vi "ELVIS III v1.0 AO Enqueue Data.vi"(7 "AO Block Channels FPGA Reference":T1, 8 "error in (no error)":errorcluster, 11 "AO Block Write Configuration":T2={"AO FIFO Clock Divisor"=1000, "Wait Until Done?"=TRUE, "Write Mode"=0, "AO (N Samples) Configuration "=[]}) -> (0 "error out":errorcluster)   [LabVIEW 2021]
uses:
  <vilib>/myRIO/Common/Instrument Driver Framework/ELVIS III v1.0/AO Block/typedefs/ELVIS III AO Block Configuration.ctl
  <vilib>/myRIO/Common/Instrument Driver Framework/ELVIS III v1.0/AO Block/typedefs/ELVIS III AO Block Bank Data.ctl
  <vilib>/myRIO/Common/Instrument Driver Framework/ELVIS III v1.0/AO Block/typedefs/ELVIS III AO Block Channels FPGA Reference.ctl
  <vilib>/rvi/errors/niLvFpgaAdjustHostInterfaceError.vi
  <vilib>/rvi/interface/nirviReadWriteControl/nirviReadWriteControl.xnode
  NiFpgaLv.dll
  <vilib>/rvi/interface/Simulation/niFpgaSimulationCallBeginRW.vi
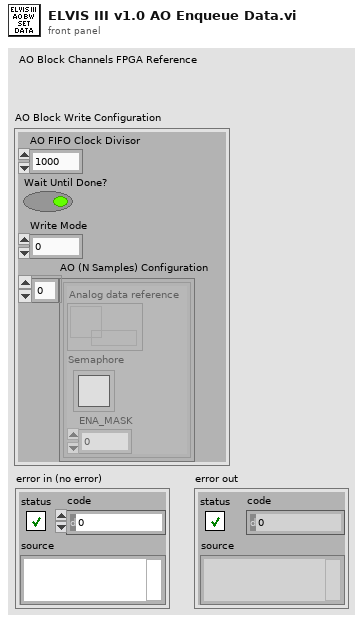
[diagram p1: front panel]
types:
  T1 = typedef "ELVIS III AO Block Channels FPGA Reference.ctl" = refnum<k20>
  T2 = typedef "ELVIS III AO Block Configuration.ctl" = cluster{"AO FIFO Clock Divisor":u32, "Wait Until Done?":bool, "Write Mode":u8, "AO (N Samples) Configuration ":T3[]}
  T3 = typedef "ELVIS III AO Block Bank Data.ctl" = cluster{"Analog data reference":refnum<data-value>, "Semaphore":T4, "ENA_MASK":u8}
  T4 = typedef "Semaphore RefNum" = refnum<k1>
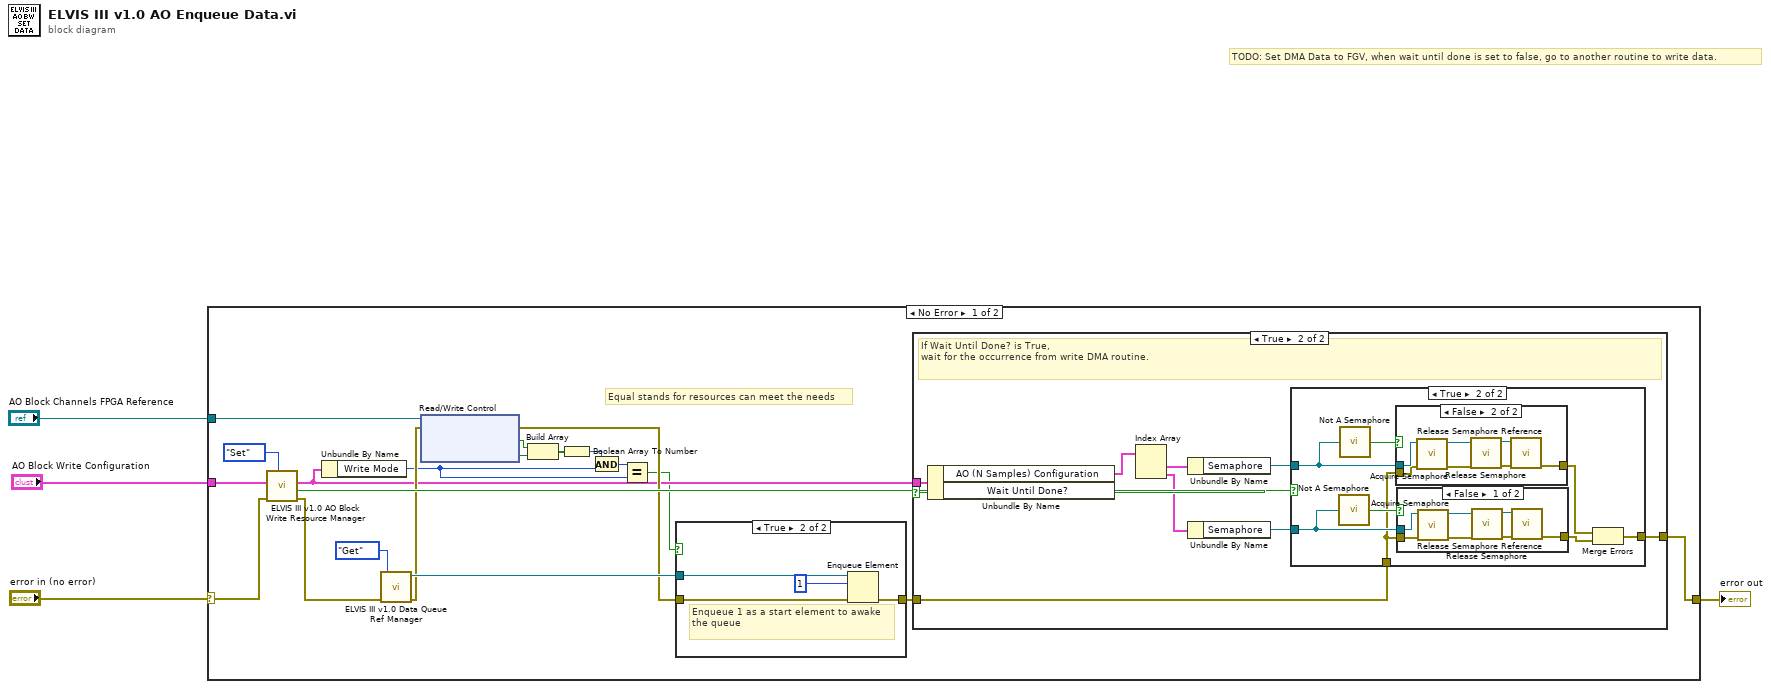
[diagram p0: block diagram]
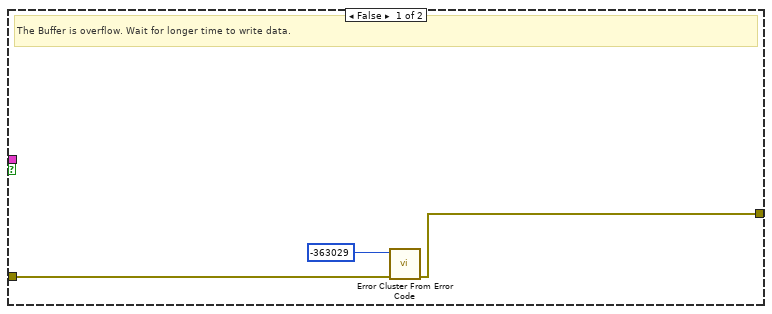
[diagram p3: hidden frame]
diagram:
  # "TODO: Set DMA Data to FGV, when wait until done is set to false, go to another routine to write data."
  n1 = case shown="No Error" "error in (no error)" {
    selector: "error in (no error)" -> [w20 w67]
    tunnel: [w5 w67] -> w3
    tunnel: "AO Block Write Configuration" -> [w6 _]
    tunnel: "AO Block Channels FPGA Reference" -> [w24 _]
    frame No Error {
      # "Equal stands for resources can meet the needs"
      n2 = call <vilib>:"ELVIS III v1.0 AO Block Write Resource Manager.vi"("Action"=enum16{"Set", "Get"}."Set", "error in (no error)"=w20, "AO Resource In"=w6) -> ("error out"=w21:errorcluster, "Action Succeeds"=w22:bool, "AO Resource Out"=w14:T2)  [unwired: 6 in]
      n3 = Unbundle By Name(w14) -> ("Write Mode"=w8:u8)
      n4 = call <vilib>:"ELVIS III v1.0 Data Queue Ref Manager.vi"("Action"=enum16{"Get", "Reset"}."Get", "error in (no error)"=w21) -> ("error out"=w16:errorcluster, "Queue out"=w18:refnum<queue>)  [unwired: 7 in]
      n5 = xnode "Read/Write Control"("FPGA VI Reference In"=w24, "error in"=w16) -> ("error out"=w15:errorcluster, "AO.A.DMA_IDL"=w13:bool, "AO.B.DMA_IDL"=w12:bool)  [unwired: 1 out]
      n6 = Build Array(w13, w12) -> (w11:bool[])
      n7 = Boolean Array To Number(Boolean array=w11) -> (number=w10:u8)
      n8 = And(x=w10, y=w8) -> (x .and. y?=w9:u8)
      n9 = Equal?(x=w9, y=w8) -> (x = y?=w7:bool)
      n10 = case shown="True" w7 {
        tunnel: w18 -> [_ w29]
        tunnel: [w25 w28] -> w23
        tunnel: w15 -> [w25 w27]
        frame False {
        }
        frame True {
          # "Enqueue 1 as a start element to awake the queue"
          n11 = Enqueue Element(queue=w29, element=1, error in (no error)=w27) -> (error out=w28:errorcluster)  [unwired: 1 in, 2 out]
        }
      }
      n12 = case shown="True" w22 {
        tunnel: w23 -> [w31 w34]
        tunnel: w14 -> [_ w40]
        tunnel: [w30 w33] -> w5
        frame False {
          # "The Buffer is overflow. Wait for longer time to write data."
          n13 = call <vilib>:"Error Cluster From Error Code.vi"("error in (no error)"=w31, "error code (0)"=-363029) -> ("error out"=w30:errorcluster)  [unwired: 7 in]
        }
        frame True {
          # "If Wait Until Done? is True, \nwait for the occurrence from write DMA routine."
          n14 = Unbundle By Name(w40) -> ("AO (N Samples) Configuration"=w39:T3[], "Wait Until Done?"=w41:bool)
          n15 = Index Array(array=w39) -> (element #1=w38:T3, element #2=w36:T3)  [unwired: 2 in]
          n16 = Unbundle By Name(w38) -> ("Semaphore"=w37:T4)
          n17 = Unbundle By Name(w36) -> ("Semaphore"=w35:T4)
          n18 = case shown="True" w41 {
            tunnel: w37 -> [_ w50]
            tunnel: w35 -> [_ w48]
            tunnel: w34 -> [w42 w46]
            tunnel: [w42 w43] -> w33
            frame False {
            }
            frame True {
              n19 = call <vilib>:"Not A Semaphore.vi"("semaphore"=w48) -> ("not a semaphore"=w47:bool)
              n20 = call <vilib>:"Not A Semaphore.vi"("semaphore"=w50) -> ("not a semaphore"=w49:bool)
              n21 = case shown="False" w49 {
                tunnel: w50 -> [_ w66]
                tunnel: w46 -> [w59 w61]
                tunnel: [w59 w60] -> w45
                frame True {
                }
                frame False {
                  n22 = call <vilib>:"Acquire Semaphore.vi"("error in (no error)"=w61, "semaphore"=w66) -> ("error out"=w65:errorcluster, "semaphore out"=w64:T4)  [unwired: 3 in, 1 out]
                  n23 = call <vilib>:"Release Semaphore.vi"("error in (no error)"=w65, "semaphore"=w64) -> ("error out"=w62:errorcluster, "semaphore out"=w63:T4)  [unwired: 4 in]
                  n24 = call <vilib>:"Release Semaphore Reference.vi"("error in (no error)"=w62, "semaphore"=w63) -> ("error out"=w60:errorcluster)  [unwired: 8 in, 1 out]
                }
              }
              n25 = case shown="False" w47 {
                tunnel: w48 -> [w55 _]
                tunnel: w46 -> [w52 w58]
                tunnel: [w51 w58] -> w44
                frame False {
                  n26 = call <vilib>:"Acquire Semaphore.vi"("error in (no error)"=w52, "semaphore"=w55) -> ("error out"=w56:errorcluster, "semaphore out"=w57:T4)  [unwired: 3 in, 1 out]
                  n27 = call <vilib>:"Release Semaphore.vi"("error in (no error)"=w56, "semaphore"=w57) -> ("error out"=w53:errorcluster, "semaphore out"=w54:T4)  [unwired: 4 in]
                  n28 = call <vilib>:"Release Semaphore Reference.vi"("error in (no error)"=w53, "semaphore"=w54) -> ("error out"=w51:errorcluster)  [unwired: 8 in, 1 out]
                }
                frame True {
                }
              }
              n29 = Merge Errors(w45, w44) -> (w43:errorcluster)
            }
          }
        }
      }
    }
    frame Error {
    }
  }
  "error out" <- w3
